vi "AM_DC_Test.vi"() -> ()   [LabVIEW 2019]
doc: "Perform DC sweep measurements using the Arduino Micro, specifically check that you can characterise a diode and an npn BJT\n\nR. Sheehan 25 - 11 - 2020"
uses:
  Arrays/Build_Array.vi
  <vilib>/Instr/_visa.llb/VISA Configure Serial Port (Instr).vi
  <vilib>/Analysis/NI_AALPro.lvlib
panel:
  in  "Tab Control":T1(tab)=enum."BJT Char"
  out "Open":bool
  out "Addr 2":refnum<visa-resource-name>="COM9"
  in  "Addr":refnum<visa-resource-name>="COM9"
  in  "Open Comms":bool
  in  "Stop":bool
  out "error out":errorcluster
  in  "Write Vout":bool
  in  "Vout / V":dbl min=0.0 max=3.3
  in  "Delay (ms)":u32=4000 min=500 max=20000 step=1
  out "Cmd":string
  in  "Nreads":i32=5 min=3 max=50 step=1
  in  "Read":bool
  out "Buffer Data":string[](array[string])
  in  "Format":bool
  out "Meas / V":dbl[](array[numeric])
  out "Err / V":dbl[](array[numeric])
  out "Buffer Size":i32
  out "Time Taken / s":dbl
  out "XY Graph":cluster{"Idata":dbl[], "Vdata":dbl[]}(graph)
  in  "Diode Char":bool
  in  "R / kOhm":dbl
  in  "Vhigh / V":dbl
  in  "Vlow / V":dbl
  in  "Vdelta / V":dbl
  out "Current":cluster{"SwpData":dbl[], "SwpData":dbl[]}(graph)={"SwpData"=[1.6690000000000005, 1.6129999999999989, 1.5570000000000006, 1.4869999999999994, 1.403428571428571, 1.3688571428571428, 1.3198571428571404, 1.3060000000000027, 1.201000000000002, 1.201000000000001, 1.1798571428571425], "SwpData"=[15.557142857142857, 21.05102040816327, 27.92857142857143, 33.7142857142857, 39.2, 44.981632653061226, 50.17142857142856, 55.16122448979591, 60.04285714285713, 64.52857142857142, 68.62857142857145]}
  in  "Vinc / V":dbl=0.1
  in  "Vlo / V":dbl=1.0
  in  "Vhi / V":dbl=2.0
  out "Rb / Rc":dbl=14.285714285714286
  in  "BJT Char":bool=TRUE
  in  "Rc / kOhm":dbl=0.007
  in  "Rb / kOhm":dbl=0.1
  in  "Vb / V":dbl=1.65
  out "IV Char":cluster{"SwpData":dbl[], "SwpData":dbl[]}(graph)={"SwpData"=[0.050300000000000004, 0.0684, 0.0831, 0.10191428571428572, 0.11729999999999999, 0.13758571428571428, 0.1599, 0.18500000000000003, 0.21510000000000004, 0.24930000000000002, 0.30860000000000004], "SwpData"=[15.557142857142857, 21.05102040816327, 27.92857142857143, 33.7142857142857, 39.2, 44.981632653061226, 50.17142857142856, 55.16122448979591, 60.04285714285713, 64.52857142857142, 68.62857142857145]}
  out "SwpData":dbl[][](array[numeric])=[[0.9412, 0.1585, 1.6690000000000005, 15.557142857142857, 0.050300000000000004], [0.9454, 0.2157571428571429, 1.6129999999999989, 21.05102040816327, 0.0684], [0.9481999999999999, 0.2786, 1.5570000000000006, 27.92857142857143, 0.0831], [0.9489, 0.3372285714285714, 1.4869999999999994, 33.7142857142857, 0.10191428571428572], [0.9489, 0.3924, 1.403428571428571, 39.2, 0.11729999999999999], [0.9509857142857143, 0.4531428571428571, 1.3688571428571428, 44.981632653061226, 0.13758571428571428], [0.9537857142857142, 0.5117999999999999, 1.3198571428571404, 50.17142857142856, 0.1599], [0.9552000000000002, 0.5718285714285714, 1.3060000000000027, 55.16122448979591, 0.18500000000000003], [0.9503, 0.6354, 1.201000000000002, 60.04285714285713, 0.21510000000000004], [0.9524, 0.701, 1.201000000000001, 64.52857142857142, 0.24930000000000002], [0.9530857142857142, 0.7883000000000001, 1.1798571428571425, 68.62857142857145, 0.30860000000000004]]
  out "beta":dbl=-103.30507075511545
  in  "BJT Swp In":T2={"Vb / V"=0.0, "Vhi / V"=0.0, "Vlo / V"=0.0, "Vinc / V"=0.0, "Rb / kOhm"=0.0, "Rc / kOhm"=0.0, "Delay (ms)"=500, "Nreads"=3} {"Nreads" min=3 max=50 step=1; "Delay (ms)" min=4000 max=20000 step=1}
  # "Vb / V"
  # "Vc / V"
  # "Ib / mA"
  # "Ic / mA"
  # "Vce / V"
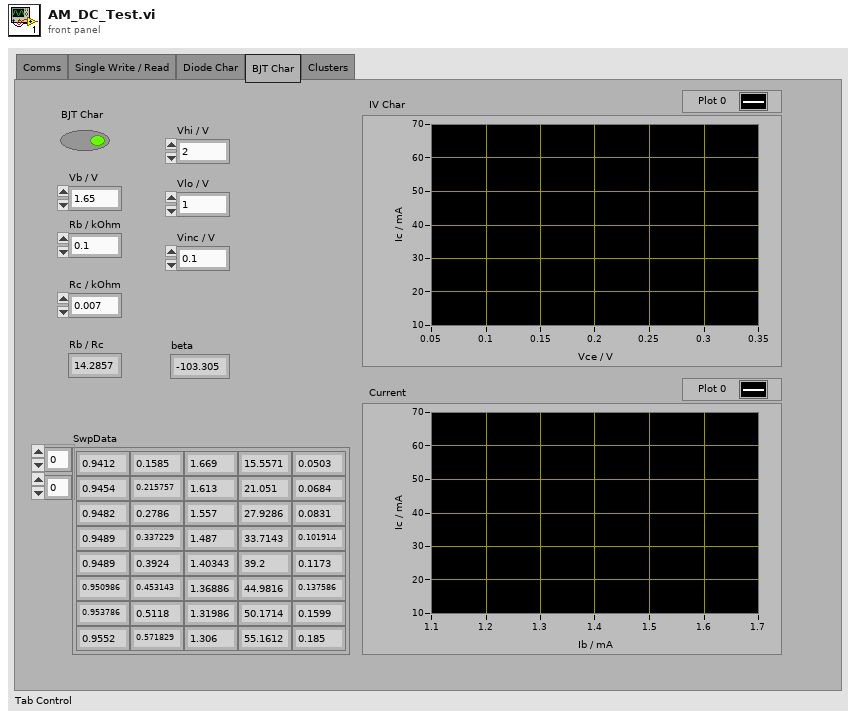
[diagram p1: front panel]
types:
  T1 = enum32{"Comms", "Single Write / Read", "Diode Char", "BJT Char", "Clusters"}
  T2 = cluster{"Vb / V":dbl, "Vhi / V":dbl, "Vlo / V":dbl, "Vinc / V":dbl, "Rb / kOhm":dbl, "Rc / kOhm":dbl, "Delay (ms)":u32, "Nreads":i32}
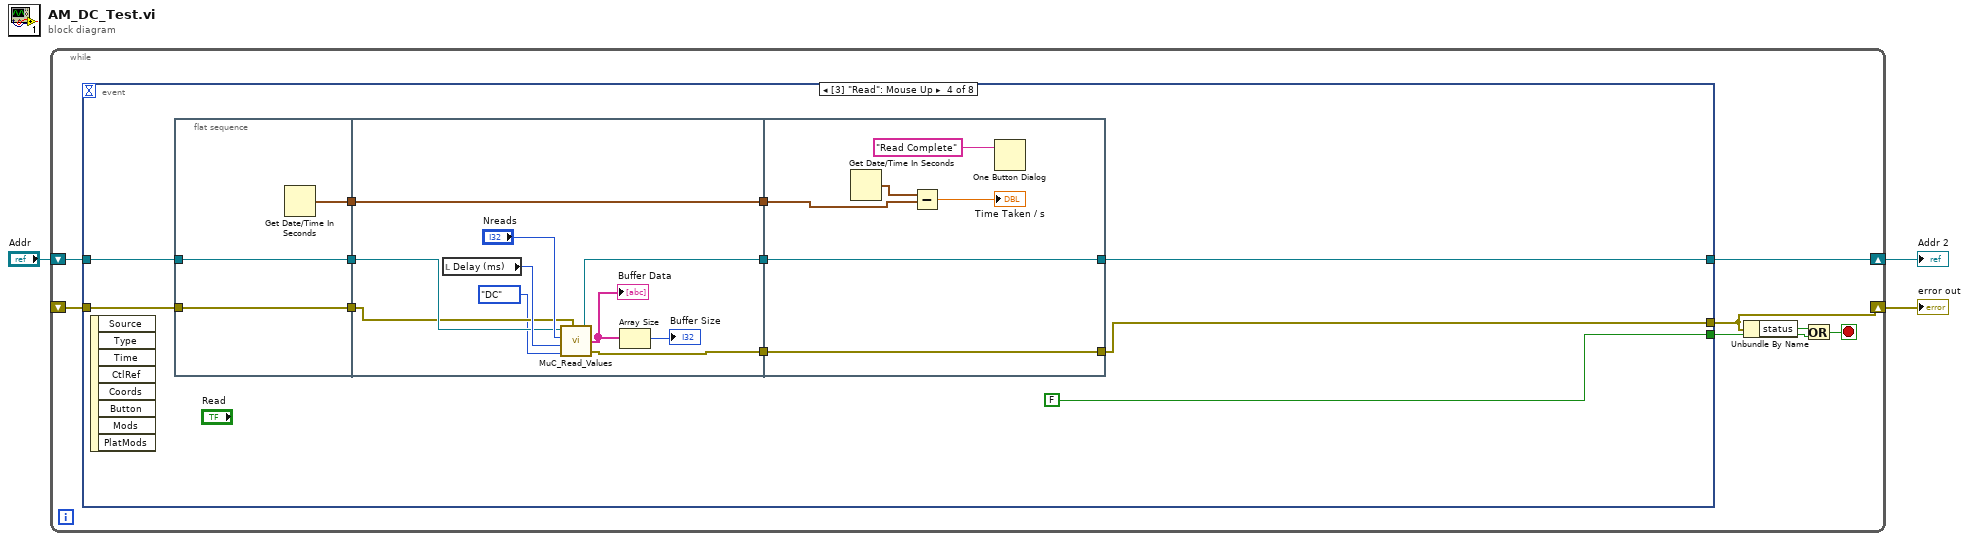
[diagram p0: block diagram]
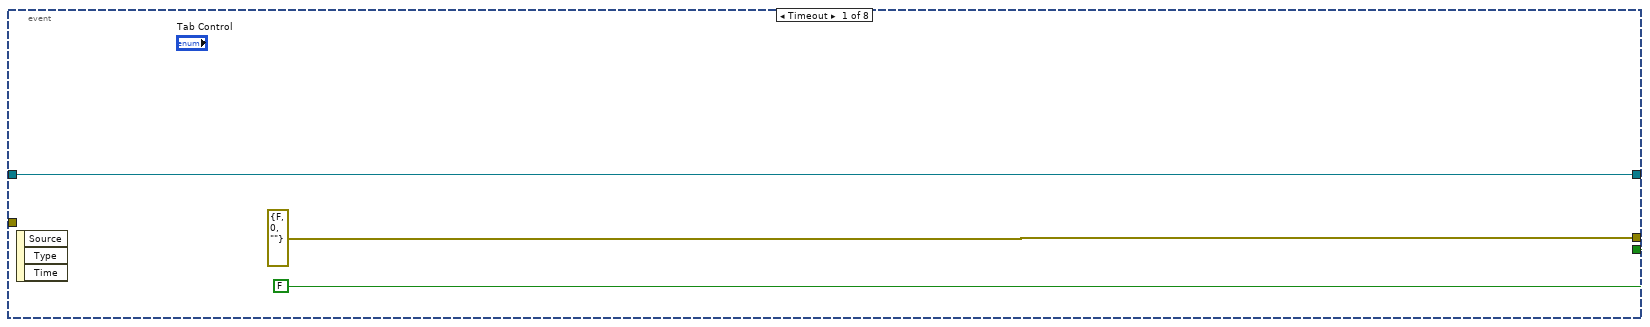
[diagram p2: hidden frame]
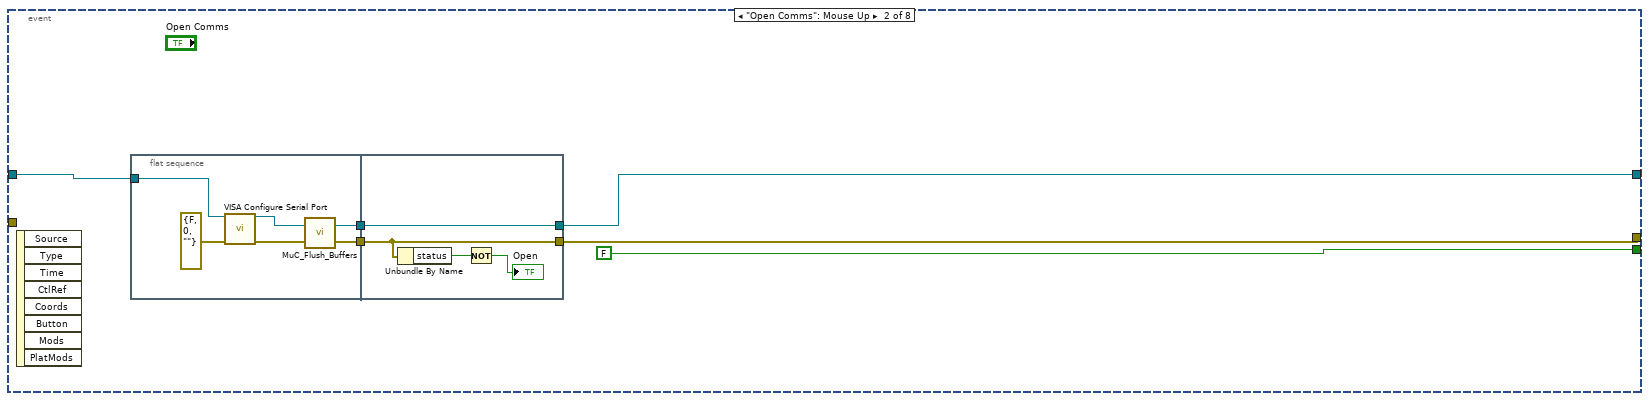
[diagram p3: hidden frame]
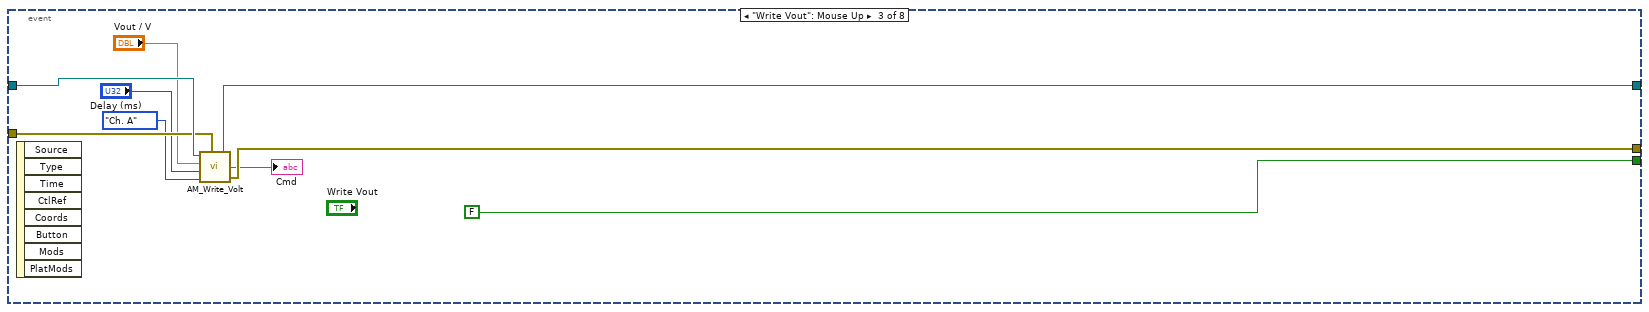
[diagram p4: hidden frame]
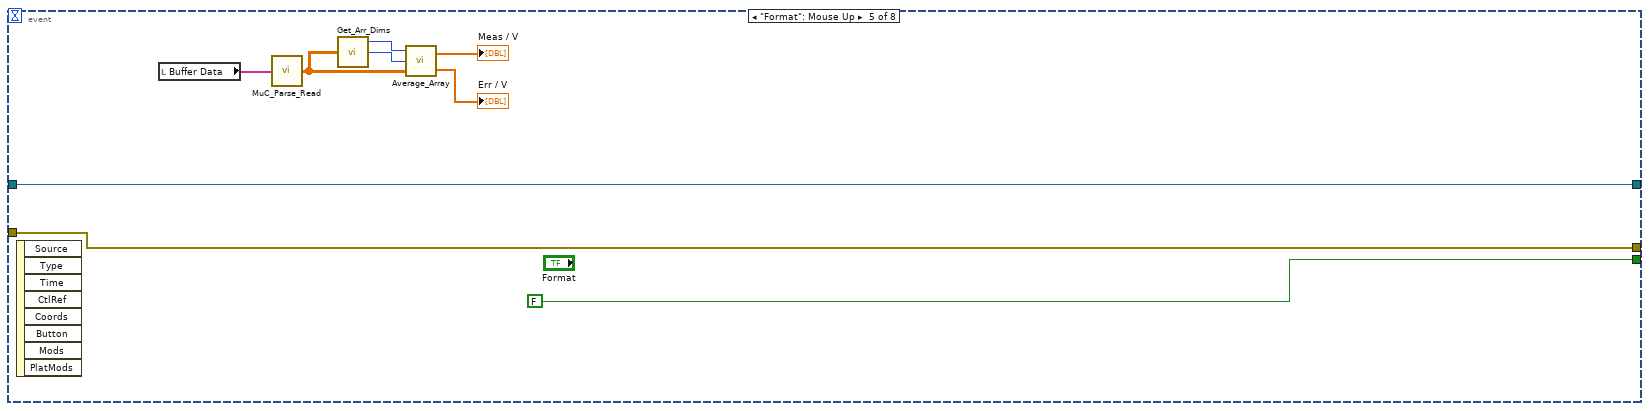
[diagram p5: hidden frame]
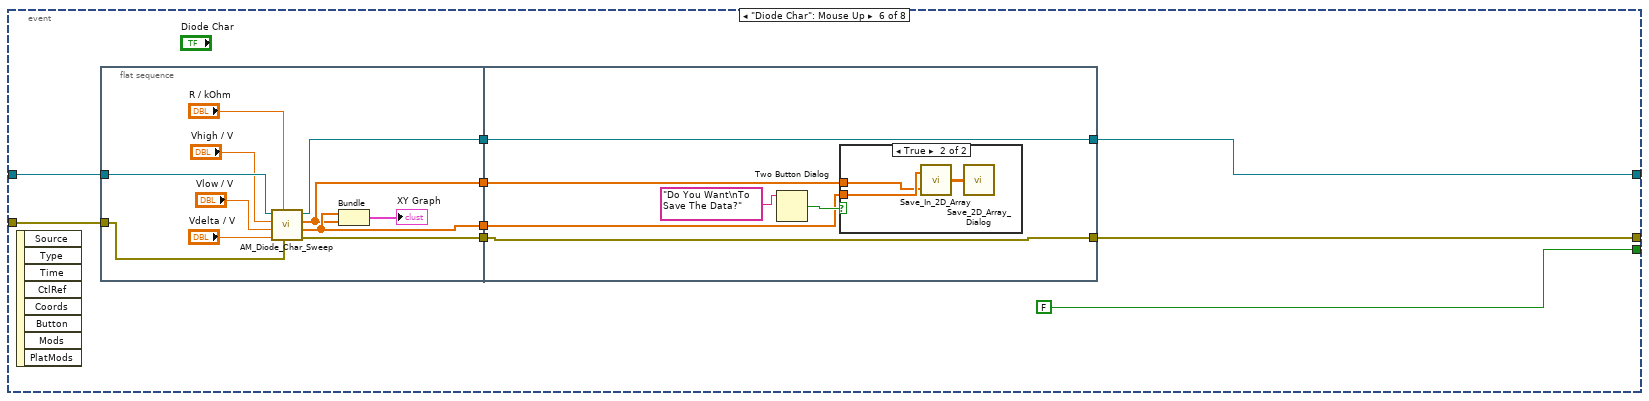
[diagram p6: hidden frame]
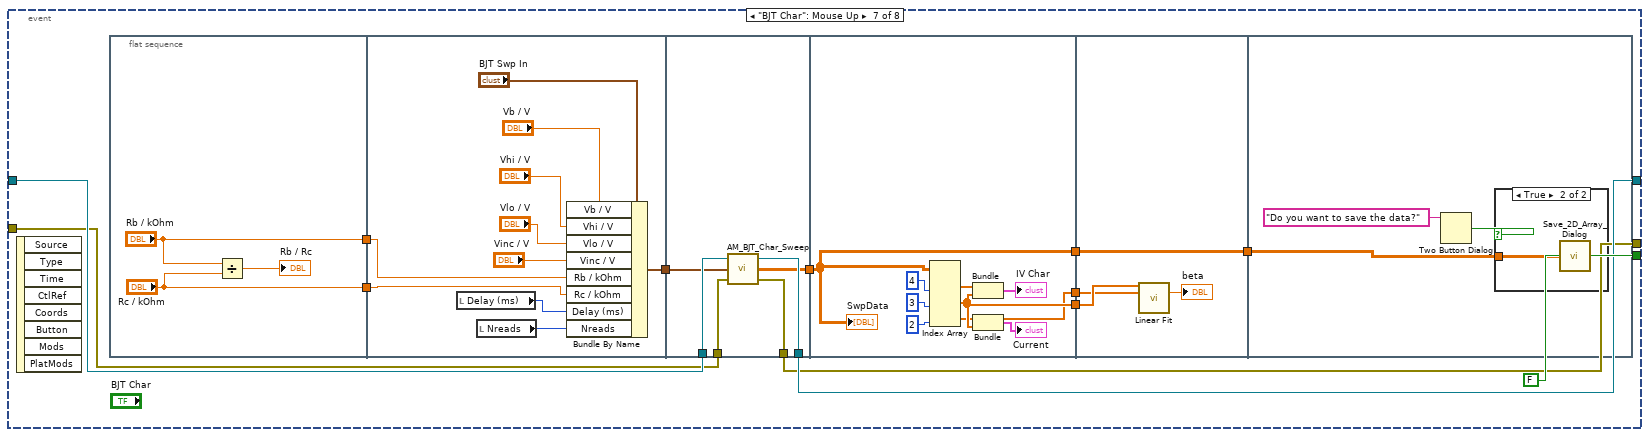
[diagram p8: hidden frame]
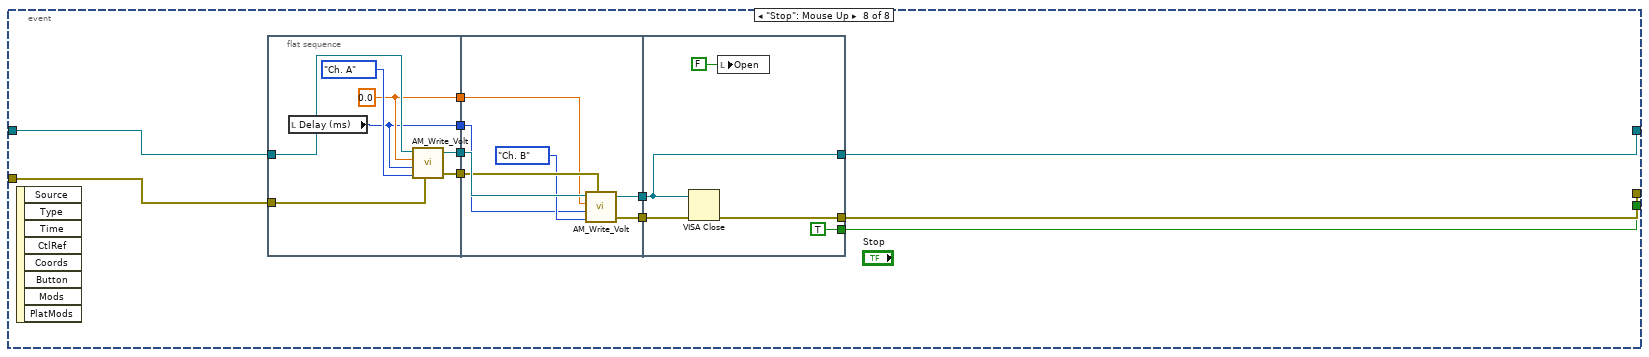
[diagram p10: hidden frame]
diagram:
  n1 = while {
    shift-right: [w9] -> w2
    shift-left: "Addr" -> [w10]
    shift-right: [w8] -> w1
    shift-left: _ -> [w7]
    stop <- w5 stop-if-true
    n2 = event shown="[3] \"Read\": Mouse Up" {
      selector: _ -> [_ _ _ _ _ _ _ _]
      dyn-events: _ -> [_ _ _ _ _ _ _ _]
      timeout: _ -> [_ _ _ _ _ _ _ _]
      tunnel: w10 -> [w11 w19 w37 w48 w77 w85 w116 w164]
      tunnel: [w11 w17 w34 w46 w77 w84 w113 w163] -> w9
      tunnel: [errorcluster {"status"=FALSE, "code"=0, "source"=""} ("error in (no error)") w14 w33 w45 w69 w83 w112 w166] -> w8
      tunnel: w7 -> [_ _ w36 w47 w69 w86 w114 w165]
      tunnel: [FALSE FALSE FALSE FALSE FALSE FALSE FALSE w156] -> w4
      event Timeout {
        n3 = event-data() -> ()  [unwired: 1 in, 3 out]
      }
      event "Open Comms": Mouse Up {
        n4 = event-data() -> ()  [unwired: 1 in, 8 out]
        n5 = flat-sequence {
          tunnel: w19 -> [w24]
          tunnel: [w22] -> w16
          tunnel: [w20] -> w15
          tunnel: [w29] -> w17
          tunnel: w16 -> [w29]
          tunnel: w15 -> [w28]
          tunnel: [w28] -> w14
          frame #0 {
            n6 = call-poly "VISA Configure Serial Port"("VISA resource name"=w24, "error in (no error)"=errorcluster {"status"=FALSE, "code"=0, "source"=""}) -> ("VISA resource name out"=w23:refnum<visa-resource-name>, "error out"=w21:errorcluster)  [unwired: 7 in, 5 out]
            n7 = call "MuC_Flush_Buffers.vi"("error in (no error)"=w21, "VISA resource name"=w23) -> ("error out"=w20:errorcluster, "VISA resource name 2"=w22:refnum<visa-resource-name>)
          }
          frame #1 {
            n8 = Unbundle By Name(w28) -> ("status"=w26:bool)
            n9 = Not(x=w26) -> (.not. x?=→"Open":bool)
          }
        }
      }
      event "Write Vout": Mouse Up {
        n10 = event-data() -> ()  [unwired: 1 in, 8 out]
        n11 = call "AM_Write_Volt.vi"("VISA resource name"=w37, "Volt / V"="Vout / V", "Delay / ms"="Delay (ms)", "Enum"=enum16{"Ch. A", "Ch. B"}."Ch. A", "error in (no error)"=w36) -> ("VISA resource name 2"=w34:refnum<visa-resource-name>, "Cmd"=→"Cmd":string, "error out"=w33:errorcluster)
      }
      event "Read": Mouse Up {
        n12 = event-data() -> ()  [unwired: 1 in, 8 out]
        n13 = flat-sequence {
          tunnel: w47 -> [w51]
          tunnel: w48 -> [w52]
          tunnel: [w52] -> w42
          tunnel: [w51] -> w41
          tunnel: [w50] -> w39
          tunnel: [w62] -> w44
          tunnel: [w61] -> w43
          tunnel: w42 -> [w56]
          tunnel: w41 -> [w55]
          tunnel: [w53] -> w40
          tunnel: w39 -> [w53]
          tunnel: [w67] -> w45
          tunnel: [w68] -> w46
          tunnel: w44 -> [w68]
          tunnel: w43 -> [w67]
          tunnel: w40 -> [w64]
          frame #0 {
            n14 = Get Date/Time In Seconds() -> (seconds since 1Jan1904=w50:timestamp)
          }
          frame #1 {
            n15 = local read "Delay (ms)"() -> (w60:u32)
            n16 = call "MuC_Read_Values.vi"("VISA resource name"=w56, "Nreads"="Nreads", "Delay (ms)"=w60, "Read Type"=enum16{"DC", "AC"}."DC", "error in (no error)"=w55) -> ("VISA resource name 2"=w62:refnum<visa-resource-name>, "Buffer Data"=w58:string[], "error out"=w61:errorcluster)
            "Buffer Data" <- w58
            n17 = Array Size(array=w58) -> (size(s)=→"Buffer Size":i32)
          }
          frame #2 {
            n18 = Get Date/Time In Seconds() -> (seconds since 1Jan1904=w65:timestamp)
            n19 = Subtract(x=w65, y=w64) -> (x-y=→"Time Taken / s":dbl)
            n20 = One Button Dialog(message="Read Complete") -> ()  [unwired: 1 in, 1 out]
          }
        }
      }
      event "Format": Mouse Up {
        n21 = event-data() -> ()  [unwired: 1 in, 8 out]
        n22 = local read "Buffer Data"() -> (w75:string[])
        n23 = call "MuC_Parse_Read.vi"("Buffer Data"=w75) -> ("Data"=w72:dbl[][])
        n24 = call "Get_Arr_Dims.vi"("Data"=w72) -> ("N Rows"=w71:i32, "N Cols"=w70:i32)  [unwired: 1 out]
        n25 = call "Average_Array.vi"("Array"=w72, "Ncolumns"=w70, "Nrows"=w71) -> ("Max-Min"=→"Err / V":dbl[], "Average"=→"Meas / V":dbl[])
      }
      event "Diode Char": Mouse Up {
        n26 = event-data() -> ()  [unwired: 1 in, 8 out]
        n27 = flat-sequence {
          tunnel: w86 -> [w97]
          tunnel: w85 -> [w96]
          tunnel: [w95] -> w81
          tunnel: [w94] -> w80
          tunnel: [w88] -> w79
          tunnel: [w87] -> w78
          tunnel: [w102] -> w83
          tunnel: [w103] -> w84
          tunnel: w81 -> [w103]
          tunnel: w80 -> [w102]
          tunnel: w79 -> [w99]
          tunnel: w78 -> [w98]
          frame #0 {
            n28 = call "AM_Diode_Char_Sweep.vi"("error in"=w97, "R / kOhm"="R / kOhm", "Vdelta / V"="Vdelta / V", "Vlow / V"="Vlow / V", "Vhigh / V"="Vhigh / V", "VISA resource name 2"=w96) -> ("error out"=w94:errorcluster, "Idata"=w88:dbl[], "Vdata"=w87:dbl[], "VISA resource name 3"=w95:refnum<visa-resource-name>)
            n29 = Bundle("Idata"=w88, "Vdata"=w87) -> (→"XY Graph":cluster{"Idata":dbl[], "Vdata":dbl[]})  [unwired: 1 in]
          }
          frame #1 {
            n30 = Two Button Dialog(message="Do You Want\nTo Save The Data?") -> (T button?=w101:bool)  [unwired: 2 in]
            n31 = case shown="True" w101 {
              tunnel: w99 -> [_ w105]
              tunnel: w98 -> [_ w104]
              frame False {
              }
              frame True {
                n32 = call "Save_In_2D_Array.vi"("Vert"=w104, "Horz"=w105) -> ("Array"=w106:dbl[][])
                n33 = call "Save_2D_Array_Dialog.vi"("2D data"=w106) -> ()
              }
            }
          }
        }
      }
      event "BJT Char": Mouse Up {
        n34 = event-data() -> ()  [unwired: 1 in, 8 out]
        n35 = flat-sequence {
          tunnel: ["Rb / kOhm"] -> w118
          tunnel: ["Rc / kOhm"] -> w117
          tunnel: w118 -> [w127]
          tunnel: w117 -> [w126]
          tunnel: [w123] -> w115
          tunnel: w116 -> [w138]
          tunnel: w115 -> [w137]
          tunnel: w114 -> [w136]
          tunnel: [w135] -> w113
          tunnel: [w134] -> w112
          tunnel: [w133] -> w111
          tunnel: w111 -> [w142]
          tunnel: [w142] -> w110
          tunnel: [w140] -> w108
          tunnel: [w139] -> w107
          tunnel: w110 -> [w151]
          tunnel: [w151] -> w109
          tunnel: w108 -> [w150]
          tunnel: w107 -> [w149]
          tunnel: w109 -> [w153]
          frame #0 {
            n36 = Divide(x="Rb / kOhm", y="Rc / kOhm") -> (x/y=→"Rb / Rc":dbl)
          }
          frame #1 {
            n37 = local read "Delay (ms)"() -> (w125:u32)
            n38 = local read "Nreads"() -> (w124:i32)
            n39 = Bundle By Name(cluster="BJT Swp In", "Vb / V"="Vb / V", "Vhi / V"="Vhi / V", "Vlo / V"="Vlo / V", "Vinc / V"="Vinc / V", "Rb / kOhm"=w127, "Rc / kOhm"=w126, "Delay (ms)"=w125, "Nreads"=w124) -> (w123:T2)
          }
          frame #2 {
            n40 = call "AM_BJT_Char_Sweep.vi"("error in (no error)"=w136, "BJT Swp In"=w137, "VISA resource name"=w138) -> ("error out"=w134:errorcluster, "SwpData"=w133:dbl[][], "VISA resource name 2"=w135:refnum<visa-resource-name>)
          }
          frame #3 {
            n41 = Index Array(array=w142, index (col) #1=4 ("disabled index (col)"), index (col) #2=3 ("index (col)"), index (col) #3=2 ("index (col)")) -> (element #1=w144:dbl[], element #2=w140:dbl[], element #3=w139:dbl[])  [unwired: 3 in]
            n42 = Bundle("SwpData"=w144, "SwpData"=w140) -> (→"IV Char":cluster{"SwpData":dbl[], "SwpData":dbl[]})  [unwired: 1 in]
            n43 = Bundle("SwpData"=w139, "SwpData"=w140) -> (→"Current":cluster{"SwpData":dbl[], "SwpData":dbl[]})  [unwired: 1 in]
            "SwpData" <- w142
          }
          frame #4 {
            n44 = call <vilib>:"Linear Fit.vi"("Y"=w150, "X"=w149) -> ("slope"=→"beta":dbl)  [unwired: 9 in, 4 out]
          }
          frame #5 {
            n45 = Two Button Dialog(message="Do you want to save the data?") -> (T button?=w152:bool)  [unwired: 2 in]
            n46 = case shown="True" w152 {
              tunnel: w153 -> [_ w155]
              frame False {
              }
              frame True {
                n47 = call "Save_2D_Array_Dialog.vi"("2D data"=w155) -> ()
              }
            }
          }
        }
      }
      event "Stop": Mouse Up {
        n48 = event-data() -> ()  [unwired: 1 in, 8 out]
        n49 = flat-sequence {
          tunnel: w165 -> [w171]
          tunnel: w164 -> [w169]
          tunnel: [w173] -> w162
          tunnel: [w172] -> w160
          tunnel: [w168] -> w158
          tunnel: [w167] -> w157
          tunnel: w162 -> [w180]
          tunnel: [w179] -> w161
          tunnel: w160 -> [w178]
          tunnel: [w177] -> w159
          tunnel: w158 -> [w175]
          tunnel: w157 -> [w174]
          tunnel: [w185] -> w166
          tunnel: w161 -> [w183]
          tunnel: [w183] -> w163
          tunnel: w159 -> [w182]
          tunnel: [TRUE] -> w156
          frame #0 {
            w168 = 0.0 ("f / Hz")
            n50 = local read "Delay (ms)"() -> (w167:u32)
            n51 = call "AM_Write_Volt.vi"("VISA resource name"=w169, "Volt / V"=w168, "Delay / ms"=w167, "Enum"=enum16{"Ch. A", "Ch. B"}."Ch. A", "error in (no error)"=w171) -> ("VISA resource name 2"=w173:refnum<visa-resource-name>, "error out"=w172:errorcluster)  [unwired: 1 out]
          }
          frame #1 {
            n52 = call "AM_Write_Volt.vi"("VISA resource name"=w180, "Volt / V"=w175, "Delay / ms"=w174, "Enum"=enum16{"Ch. A", "Ch. B"}."Ch. B", "error in (no error)"=w178) -> ("VISA resource name 2"=w179:refnum<visa-resource-name>, "error out"=w177:errorcluster)  [unwired: 1 out]
          }
          frame #2 {
            n53 = VISA Close(VISA resource name=w183, error in (no error)=w182) -> (error out=w185:errorcluster)
            n54 = local write "Open"(FALSE) -> ()
          }
        }
      }
    }
    n55 = Unbundle By Name(w8) -> ("status"=w6:bool)
    n56 = Or(x=w6, y=w4) -> (x .or. y?=w5:bool)
  }
  "Addr 2" <- w2
  "error out" <- w1
